vi "Add Autosort OK pressed.vi"(0 "Ring in":refnum<vi>, 1 "Default":bool, 2 "Data OUT":T1={"Impulse Positions"=[], "No. Imp"=0, "Parameter Time Series"=[], "Parameter Impuls Series"=[], "Experiment Parameters"={"Freq"=0.0, "Vel"=0, "Acc"=0, "Stimulus"=""}, "Autosort File"=refnum, "Data File"={"Data Channels"=[], "Sample Rate"=0, "Channel List"=[]}, "Experiment data path"=path "", "Image data path"=path "", "LVS data path"=path "", "Raw copy path"=path "", "filename"="", "desaccading parameters"={"Tolerance"=0, "Acc Range"=0.0, "Sample Rate"=0, "Impulse Plane 2"=enum."Other", "Impulse dir"=FALSE}, "Experiment Parameters 2"={"Subject"="", "Strain"="", "Rotation plane"="", "Experimenter"="", "Trial"=0.0, "Time"=0.0}, "Excel"={"Excel._Application"=refnum, "Use Excel"=FALSE, "Worksheet SINE"=refnum, "Row SINE"=0, "Worksheet TRANS"=refnum, "Row TRANS"=0}, "Session Config File"=refnum, "Autosort Parameter Set"=0, "EMA Version"="", "desacc "={"Threshold 1 [Acc]"=0.0, "Threshold 2 [% of TH1]"=0, "tolerance"=0, "Search WD "=0.0, " always use TH2"=FALSE, "Range"=0.0, "Max time"=0.0, "Min time"=0.0, "Velocity Threshold"=0}, "Cycle Nr for Saccades"={"POS"=0, "NEG"=0}, "calibration name"="No file selected"} {"Parameter Time Series"."time offset" format="%.3f"; "Parameter Time Series"."Gain" format="%.1f"; "Parameter Time Series"."Offset" format="%.1f"; "Parameter Time Series"."List 1" items=["Motor-Pos", "Motor-Vel", "Lx Position-in-Head", "Ly Position-in-Head", "Lz Position-in-Head", "Lx Velocity-in-Head", "Ly Velocity-in-Head", "Lz Velocity-in-Head", "Ll Velocity-in-Head", "Lr Velocity-in-Head", "Lx Accel-in-Head", "Ly Accel-in-Head", "Lz Accel-in-Head", "Rx Position-in-Head", "Ry Position-in-Head", "Rz Position-in-Head", "Rx Velocity-in-Head", "Ry Velocity-in-Head", "Rz Velocity-in-Head", "Rl Velocity-in-Head", "Rr Velocity-in-Head", "Rx Accel-in-Head", "Ry Accel-in-Head", "Rz Accel-in-Head", "Global Trigger", "", "", ""]; "Parameter Impuls Series"."Gain" format="%.1f"; "Parameter Impuls Series"."Offset" format="%.1f"}, 5 "Str Refnum":refnum<vi>, 7 "reference 5":refnum<vi>, 9 "reference":refnum<vi>, 12 "reference 2":refnum<vi>, 13 "reference 3":refnum<vi>, 14 "reference 4":refnum<vi>) -> ()   [LabVIEW 2016]
uses:
  type-defs/TD_Statemachine-Data.ctl
  type-defs/TD_Time Series.ctl
  type-defs/TD_Impulse Parameter.ctl
  plugins/Mars 3D/Mars3D_autosort.vi
  core.lvlib
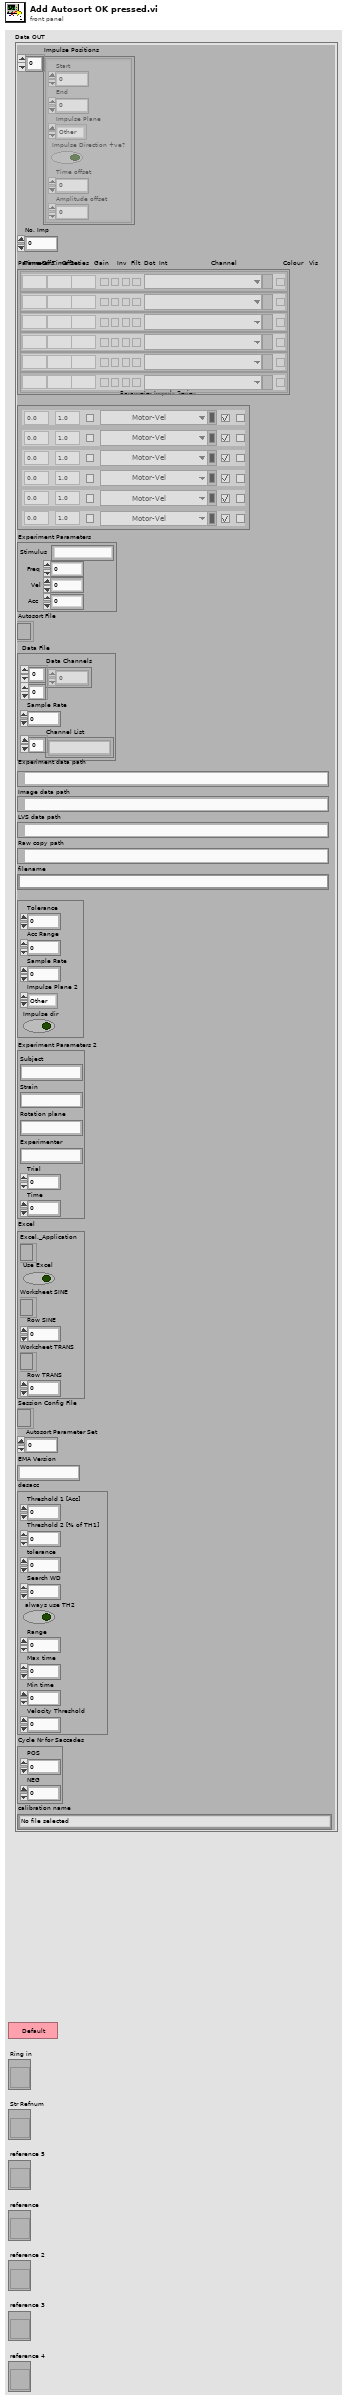
[diagram p1: front panel]
types:
  T1 = typedef "core.lvlib/TD_Statemachine-Data.ctl" = cluster{"Impulse Positions":cluster{"Start":i32, "End":i32, "Impulse Plane":enum16{"Other", "Yaw", "Pitch", "Roll", "LARP", "RALP"}, "Impulse Direction +ve?":bool, "Time offset":i32, "Amplitude offset":dbl}[], "No. Imp":i32, "Parameter Time Series":T2, "Parameter Impuls Series":T3, "Experiment Parameters":cluster{"Freq":dbl, "Vel":i32, "Acc":i32, "Stimulus":string}, "Autosort File":refnum<file>, "Data File":cluster{"Data Channels":dbl[][], "Sample Rate":i32, "Channel List":string[]}, "Experiment data path":path, "Image data path":path, "LVS data path":path, "Raw copy path":path, "filename":string, "desaccading parameters":cluster{"Tolerance":i32, "Acc Range":dbl, "Sample Rate":i32, "Impulse Plane 2":enum16{"Other", "Yaw", "Pitch", "Roll", "LARP", "RALP"}, "Impulse dir":bool}, "Experiment Parameters 2":cluster{"Subject":string, "Strain":string, "Rotation plane":string, "Experimenter":string, "Trial":dbl, "Time":dbl}, "Excel":cluster{"Excel._Application":refnum<k7>, "Use Excel":bool, "Worksheet SINE":refnum<k7>, "Row SINE":i32, "Worksheet TRANS":refnum<k7>, "Row TRANS":i32}, "Session Config File":refnum<file>, "Autosort Parameter Set":i32, "EMA Version":string, "desacc ":cluster{"Threshold 1 [Acc]":dbl, "Threshold 2 [% of TH1]":i32, "tolerance":i32, "Search WD ":dbl, " always use TH2":bool, "Range":dbl, "Max time":dbl, "Min time":dbl, "Velocity Threshold":i32}, "Cycle Nr for Saccades":cluster{"POS":i32, "NEG":i32}, "calibration name":string}
  T2 = typedef "core.lvlib/TD_Time Series.ctl" = cluster{"time offset":dbl, "Offset":dbl, "Gain":dbl, "inverse":bool, "filter data":bool, "dots":bool, "interpolate":bool, "List 1":u16, "Color Box":u32, "Boolean":bool}[]
  T3 = typedef "core.lvlib/TD_Impulse Parameter.ctl" = cluster{"Color":u32, "Visible":bool, "Channel":u16, "Invert":bool, "Desaccade":bool, "Offset":dbl, "Gain":dbl}[]
  T4 = cluster{"Min Vel /Trigger":dbl, "Width / Offset (ms)":i32, "Maximum Velocity":dbl}
  T5 = cluster{"Pre Impulse (ms)":i32, "Post Impulse (ms) ":i32, "Pitch:Roll Vel \nfor RALP/LARP ":dbl}
  T6 = cluster{"Autosize Parameter Set 2":cluster{"Trigger Ch":i32, "Min Vel":dbl, "MaxVel":dbl, "Width":i32, "Pre Impuls":i32, "Post Impuls":i32, "Pitch":dbl, "Name":string, "Other Trigger":bool, "Cross Corr":bool, "Default":cluster{"Freq":dbl, "Vel":dbl, "Acc":dbl, "Stimulus":string}}[]}[]
  T7 = cluster{"Autosize Parameter Set 2":cluster{"Trigger Ch":i32, "Min Vel":dbl, "MaxVel":dbl, "Width":i32, "Pre Impuls":i32, "Post Impuls":i32, "Pitch":dbl, "Name":string, "Other Trigger":bool, "Cross Corr":bool, "Default":cluster{"Freq":dbl, "Vel":dbl, "Acc":dbl, "Stimulus":string}}[]}
  T8 = cluster{"Trigger Ch":i32, "Min Vel":dbl, "MaxVel":dbl, "Width":i32, "Pre Impuls":i32, "Post Impuls":i32, "Pitch":dbl, "Name":string, "Other Trigger":bool, "Cross Corr":bool, "Default":cluster{"Freq":dbl, "Vel":dbl, "Acc":dbl, "Stimulus":string}}[]
  T9 = cluster{"Trigger Ch":i32, "Min Vel":dbl, "MaxVel":dbl, "Width":i32, "Pre Impuls":i32, "Post Impuls":i32, "Pitch":dbl, "Name":string, "Other Trigger":bool, "Cross Corr":bool, "Default":cluster{"Freq":dbl, "Vel":dbl, "Acc":dbl, "Stimulus":string}}
  T10 = cluster{"Freq":dbl, "Vel":i32, "Acc":i32, "Stimulus":string}
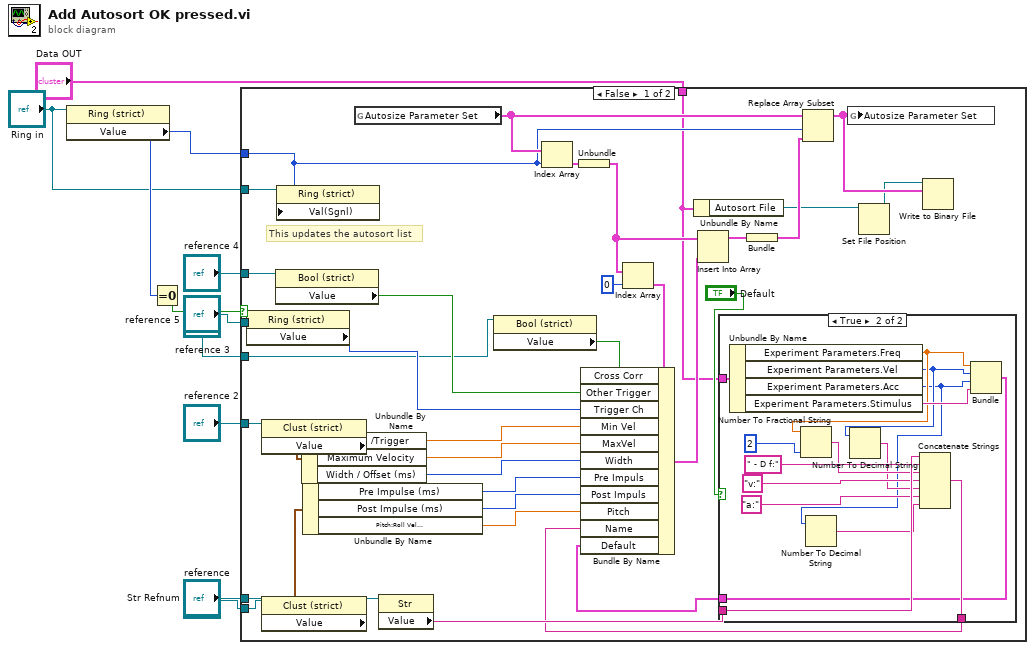
[diagram p0: block diagram]
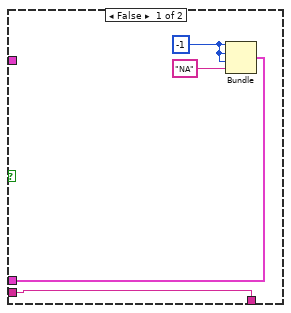
[diagram p2: hidden frame]
diagram:
  n1 = property on="Property Node" class="Ring (strict)"(reference="Ring in") -> ("Value"=w9:i8)  [unwired: 1 in, 2 out]
  n2 = Equal To 0?(x=w9) -> (x = 0?=w8:bool)
  n3 = case shown="False" w8 {
    tunnel: w9 -> [w31 _]
    tunnel: "Data OUT" -> [w21 _]
    tunnel: "Str Refnum" -> [w17 _]
    tunnel: "reference" -> [w16 _]
    tunnel: "reference 2" -> [w15 _]
    tunnel: "reference 3" -> [w14 _]
    tunnel: "Ring in" -> [w13 _]
    tunnel: "reference 4" -> [w12 _]
    tunnel: "reference 5" -> [w11 _]
    frame False {
      # "This updates the autosort list"
      n4 = property on="Property Node" class="Ring (strict)"(reference=w14) -> ("Value"=w27:u16)  [unwired: 1 in, 2 out]
      n5 = property on="Property Node" class="Clust (strict)"(reference=w15) -> ("Value"=w42:T4)  [unwired: 1 in, 2 out]
      n6 = property on="Property Node" class="Clust (strict)"(reference=w16) -> ("Value"=w41:T5)  [unwired: 1 in, 2 out]
      n7 = property class="Bool (strict)"(reference=w12) -> ("Value"=w28:bool)  [unwired: 1 in, 2 out]
      n8 = property on="Property Node" class="Ring (strict)"(reference=w13, "Val(Sgnl)"=w31) -> ()  [unwired: 1 in, 2 out]
      n9 = Unbundle By Name(w42) -> ("Min Vel /Trigger"=w37:dbl, "Maximum Velocity"=w36:dbl, "Width / Offset (ms)"=w35:i32)
      n10 = Unbundle By Name(w41) -> ("Pre Impulse (ms)"=w38:i32, "Post Impulse (ms)"=w39:i32, "Pitch:Roll Vel \nfor RALP/LARP"=w40:dbl)
      n11 = global read "Mars3D_autosort.vi" "Autosize Parameter Set"() -> (w43:T6)
      n12 = property on="Property Node" class="Str"(reference=w17) -> ("Value"=w20:string)  [unwired: 1 in, 2 out]
      n13 = property class="Bool (strict)"(reference=w11) -> ("Value"=w25:bool)  [unwired: 1 in, 2 out]
      n14 = Index Array(array=w43, index=w31) -> (element=w34:T7)
      n15 = Unbundle(w34) -> ("Autosize Parameter Set 2"=w29:T8)
      n16 = Index Array(array=w29, index=0) -> (element=w44:T9)
      n17 = Unbundle By Name(w21) -> ("Autosort File"=w24:refnum<file>)
      n18 = case shown="True" "Default" {
        tunnel: w21 -> [_ w64]
        tunnel: w20 -> [w47 w62]
        tunnel: [w47 w61] -> w19
        tunnel: [w46 w51] -> w18
        frame False {
          w49 = -1
          n19 = Bundle(w49, w49, w49, "NA") -> (w46:cluster{i32, i32, i32, string})  [unwired: 1 in]
        }
        frame True {
          n20 = Unbundle By Name(w64) -> ("Experiment Parameters.Freq"=w59:dbl, "Experiment Parameters.Vel"=w56:i32, "Experiment Parameters.Acc"=w53:i32, "Experiment Parameters.Stimulus"=w63:string)
          n21 = Number To Fractional String(number=w59, precision (6)=i16 2) -> (F-format string=w58:string)  [unwired: 2 in]
          n22 = Number To Decimal String(number=w53) -> (decimal integer string=w52:string)  [unwired: 1 in]
          n23 = Number To Decimal String(number=w56) -> (decimal integer string=w55:string)  [unwired: 1 in]
          n24 = Concatenate Strings(w62, " - D f:", w58, "v:" ("string"), w55, "a:" ("string"), w52) -> (w61:string)
          n25 = Bundle("Freq"=w59, "Vel"=w56, "Acc"=w53, "Stimulus"=w63) -> (w51:T10)  [unwired: 1 in]
        }
      }
      n26 = Bundle By Name(cluster=w44, "Cross Corr"=w25, "Other Trigger"=w28, "Trigger Ch"=w27, "Min Vel"=w37, "MaxVel"=w36, "Width"=w35, "Pre Impuls"=w38, "Post Impuls"=w39, "Pitch"=w40, "Name"=w19, "Default"=w18) -> (w33:T9)
      n27 = Insert Into Array(array=w29, new element=w33) -> (w32:T8)  [unwired: 1 in]
      n28 = Bundle("Autosize Parameter Set 2"=w32) -> (w30:T7)  [unwired: 1 in]
      n29 = Replace Array Subset(array=w43, new element=w30, index=w31) -> (w26:T6)
      n30 = global write "Mars3D_autosort.vi" "Autosize Parameter Set"(w26) -> ()
      n31 = Set File Position(refnum=w24) -> (refnum out=w23:refnum<file>)  [unwired: 3 in, 1 out]
      n32 = Write to Binary File(file (use dialog)=w23, data=w26) -> ()  [unwired: 4 in, 3 out]
    }
    frame True {
    }
  }
